vi "Result.Prompt for Comment.vi"(8 "error in (no error)":errorcluster, 11 "Comment In":string) -> (0 "error out":errorcluster, 3 "Comment Out":string)   [LabVIEW 2019]
uses:
  <vilib>/event_ctls.llb/eventvkey.ctl
panel:
  in  "Tab Control":enum32{"Inputs", "Prompt", "Outputs"}(tab)=enum."Prompt"
  in  "Comment":string
  in  "OK":bool
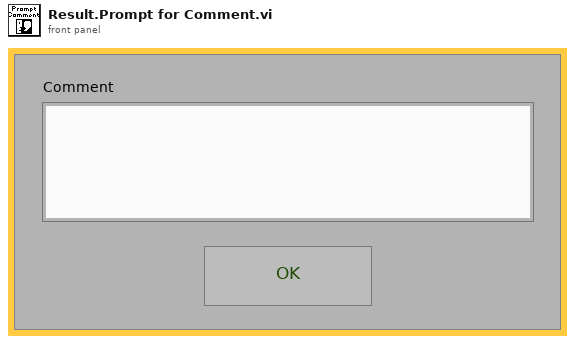
[diagram p1: front panel]
types:
  T1 = typedef "eventvkey.ctl" = enum16{"ASCII", "Enter", "Return", "Shift", "Ctrl", "Alt", "Cmd", "Opt", "Caps", "NumLock", "Clear", "Break", "Up", "Down", "Left", "Right", "Insert", "Delete", "Home", "End", "PageUp", "PageDown", "Escape", "Help", "Pause", "ScrollLock", "F1", "F2", "F3", "F4", "F5", "F6", "F7", "F8", "F9", "F10", "F11", "F12", "F13", "F14", "F15", "F16", "F17", "F18", "F19", "F20", "F21", "F22", "F23", "F24", "Play", "VolumeUp", "VolumeDown", "Mute", "Two Byte Char"}
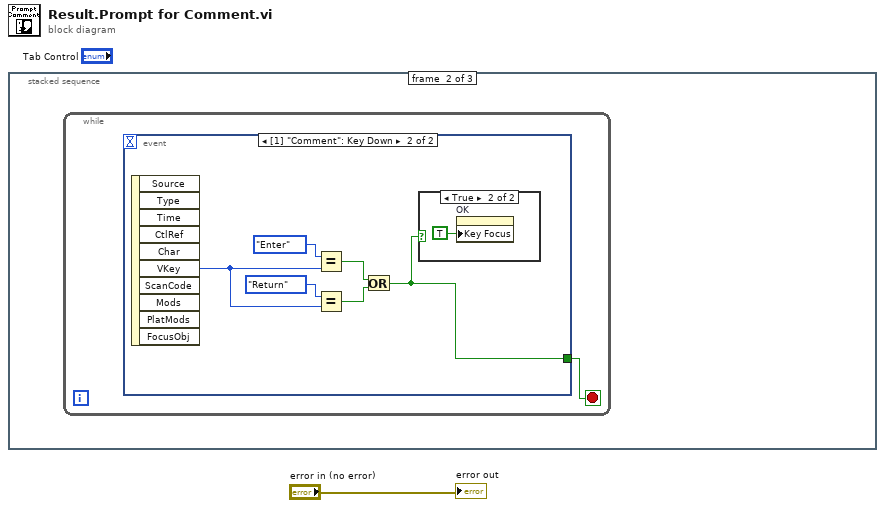
[diagram p0: block diagram]
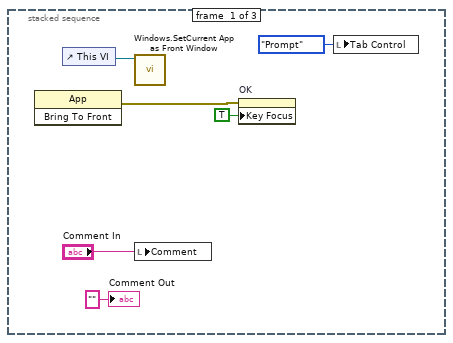
[diagram p2: hidden frame]
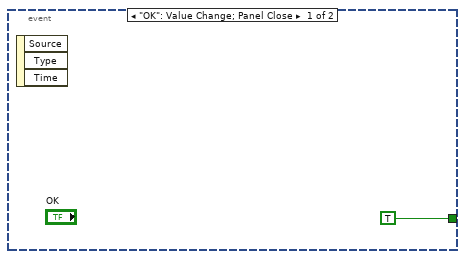
[diagram p3: hidden frame]
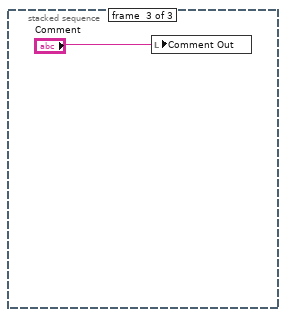
[diagram p5: hidden frame]
diagram:
  n1 = stacked-sequence {
    frame #0 {
      n2 = invoke class="App" method="Bring To Front"() -> (error out=w5:errorcluster)  [unwired: 3 in, 2 out]
      n3 = control-ref of="This VI"() -> (w7:refnum<vi>)
      n4 = call "Windows.SetCurrent App as Front Window.vi"("VI Ref"=w7) -> ()  [unwired: 11 in]
      n5 = local write "Comment"("Comment In") -> ()
      n6 = property on="OK" class="Bool"(error in=w5, "Key Focus"=TRUE) -> ()  [unwired: 1 in, 2 out]
      n7 = local write "Tab Control"(enum32{"Inputs", "Prompt", "Outputs"}."Prompt" ("Tab Control")) -> ()
      "Comment Out" <- "" ("Comment Out")
    }
    frame #1 {
      n8 = while {
        stop <- w8 stop-if-true
        n9 = event shown="[1] \"Comment\": Key Down" {
          selector: _ -> [_ _]
          dyn-events: _ -> [_ _]
          timeout: _ -> [_ _]
          tunnel: [TRUE w10] -> w8
          event "OK": Value Change; Panel Close {
            n10 = event-data() -> ()  [unwired: 1 in, 3 out]
          }
          event "Comment": Key Down {
            n11 = event-data() -> ("VKey"=w13:T1)  [unwired: 1 in, 9 out]
            n12 = Equal?(x=eventvkey."Enter" ("VKey"), y=w13) -> (x = y?=w12:bool)
            n13 = Equal?(x=eventvkey."Return" ("VKey"), y=w13) -> (x = y?=w11:bool)
            n14 = Or(x=w12, y=w11) -> (x .or. y?=w10:bool)
            n15 = case shown="True" w10 {
              frame False {
              }
              frame True {
                n16 = property on="OK" class="Bool"("Key Focus"=TRUE) -> ()  [unwired: 2 in, 2 out]
              }
            }
          }
        }
      }
    }
    frame #2 {
      (unwired) FALSE ("SelActive")
      n17 = local write "Comment Out"("Comment") -> ()
    }
  }
  "error out" <- "error in (no error)"
